vi "HGF_SVCommand.appendData2Variant.vi"(2 "error in (no error)":errorcluster, 3 "shared variable refnum":refnum<k21>, 4 "typeDescriptor":string, 5 "initData":variant) -> (0 "error out":errorcluster, 1 "dup initData":variant)   [LabVIEW 2012, in "HGF_SV.lvlib" / "HGF_SVCommand.lvclass"]
uses:
  HGF_SVCommand.lvclass
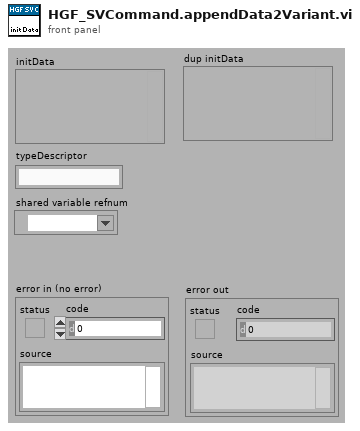
[diagram p1: front panel]
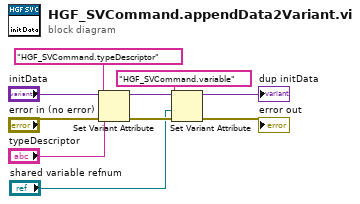
[diagram p0: block diagram]
diagram:
  n1 = Set Variant Attribute(Variant="initData", name="HGF_SVCommand.typeDescriptor", value="typeDescriptor", error in="error in (no error)") -> (Variant out=w6:variant, error out=w4:errorcluster)  [unwired: 1 out]
  n2 = Set Variant Attribute(Variant=w6, name="HGF_SVCommand.variable", value="shared variable refnum", error in=w4) -> (Variant out=→"dup initData":variant, error out=→"error out":errorcluster)  [unwired: 1 out]
